vi "短信通知设置.vi"() -> ()   [LabVIEW 2017]
uses:
  <vilib>/Utility/xml.llb/Write to XML File(string).vi
panel:
  in  "通讯录菜单":enum16{"添加", "删除"}(ring)
  in  "联系人数组":cluster{"姓名":string, "手机号":string}[](array[cluster])
  in  "密码":string
  in  "短信通道":string
  in  "员工编号":string
  in  "企业编号":string
  in  "确定":bool
  in  "取消":bool
  in  "添加联系人":bool
  in  "通讯录":i32(listbox)
  # "登录信息"
  # "通讯录"
  # "* 短信通知功能需用户自行开通，详询对接平台 http://www.c123.com/"
  # "* 通讯录表格中右键菜单添加或删除联系人"
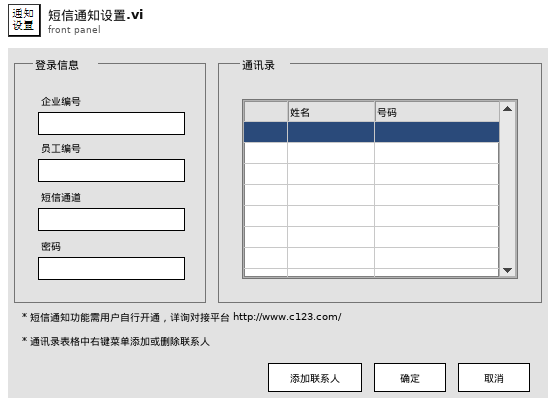
[diagram p1: front panel]
types:
  T1 = enum32{"Invalid", "Standard", "Closed", "Hidden", "Minimized", "Maximized"}
  T2 = cluster{"企业编号":string, "员工编号":string, "通道号":string, "密码":string, "联系人数组":cluster{"姓名":string, "手机号":string}[]}
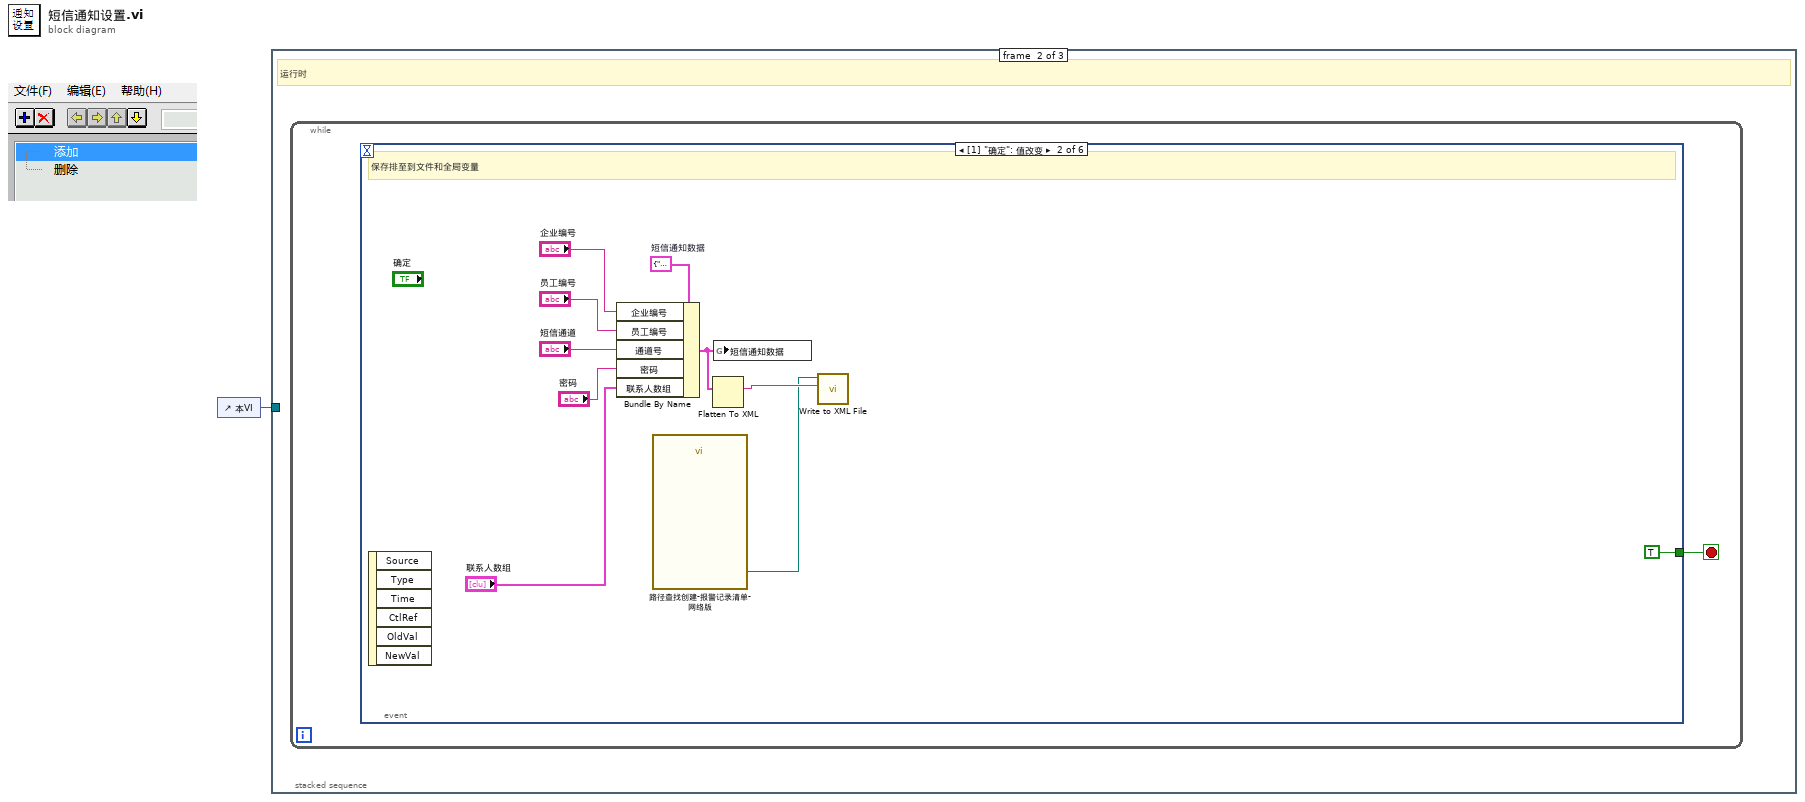
[diagram p0: block diagram]
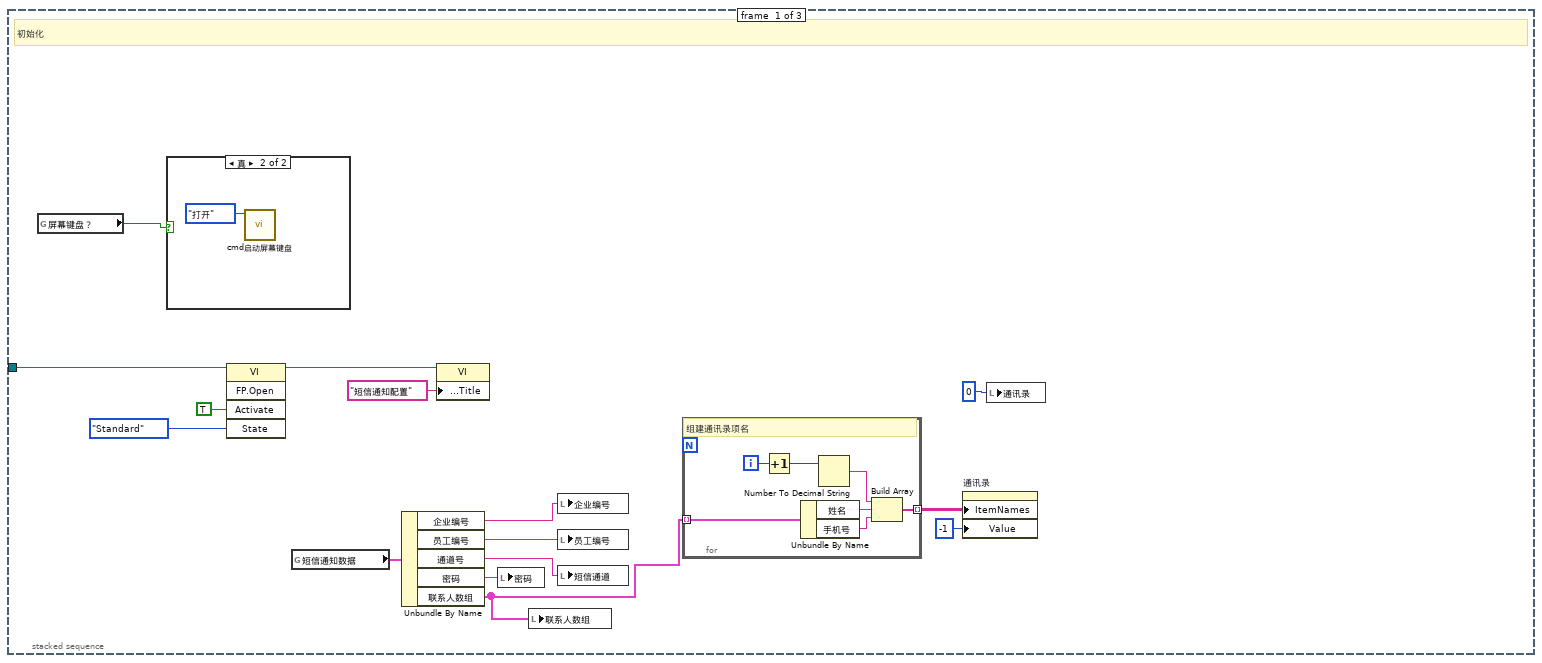
[diagram p2: hidden frame]
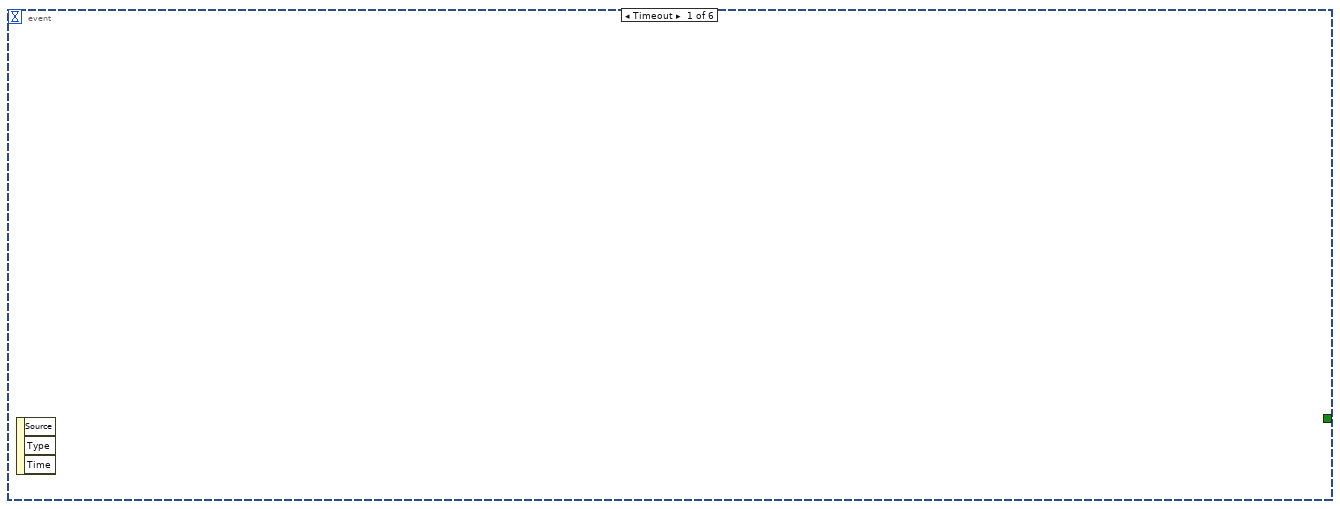
[diagram p4: hidden frame]
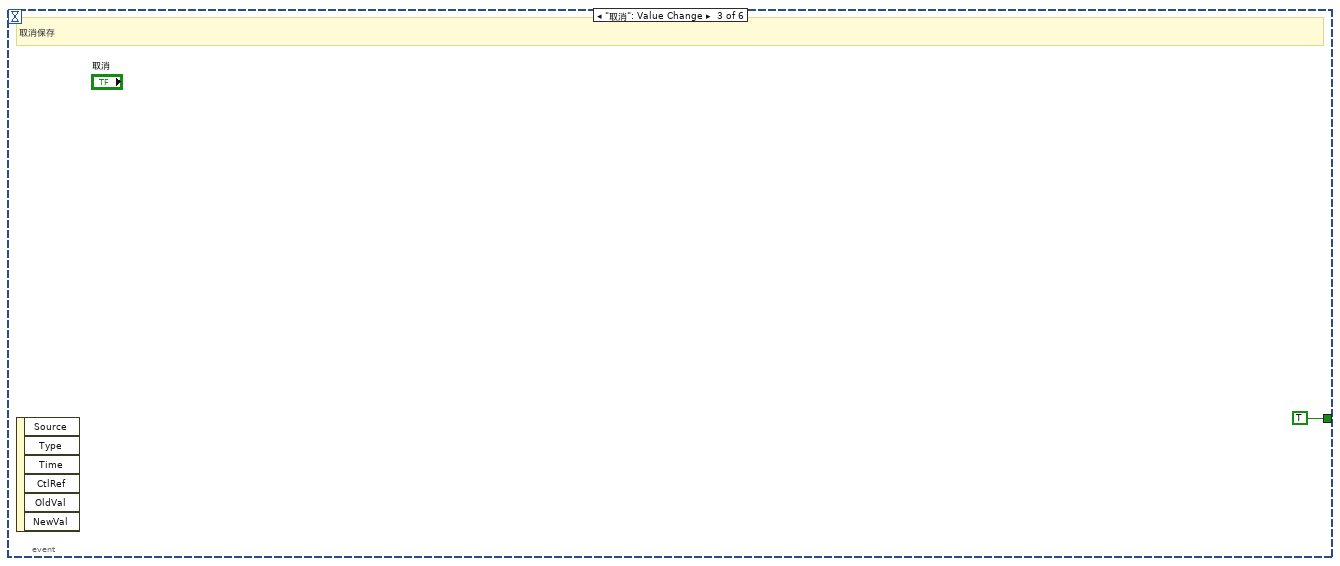
[diagram p5: hidden frame]
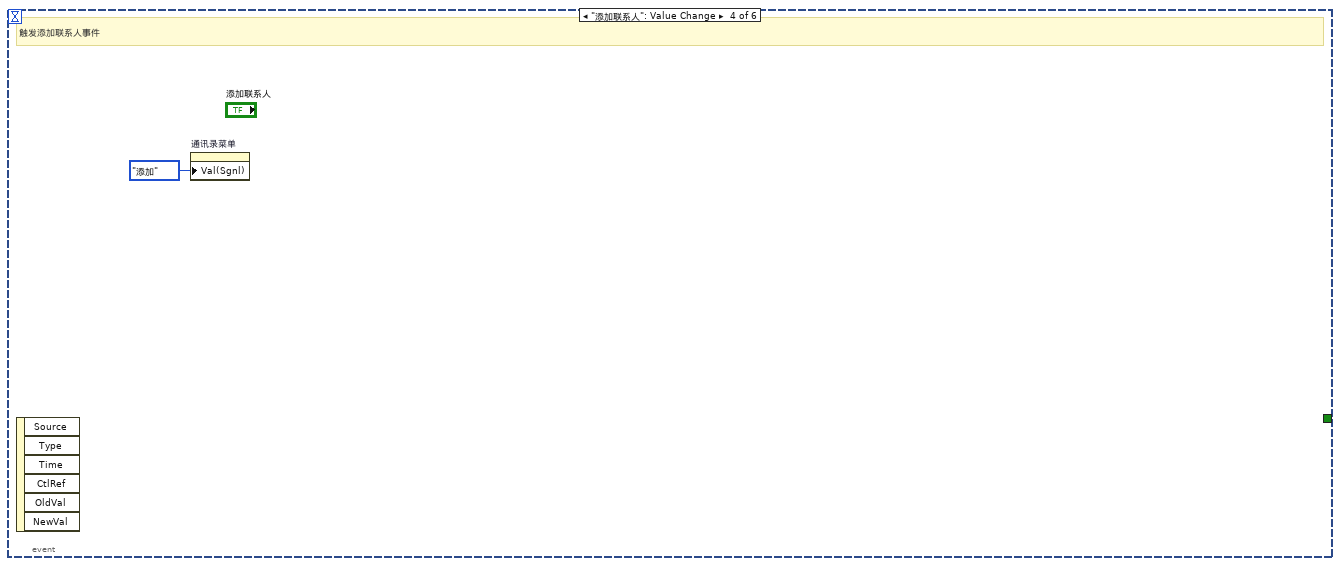
[diagram p6: hidden frame]
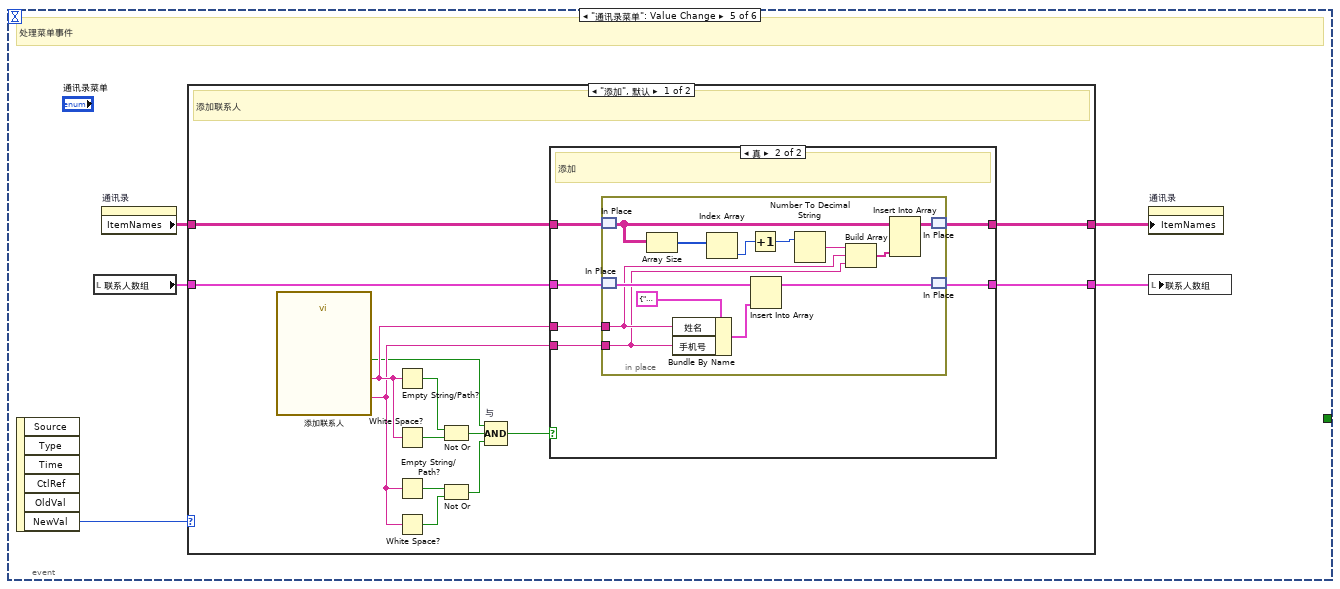
[diagram p7: hidden frame]
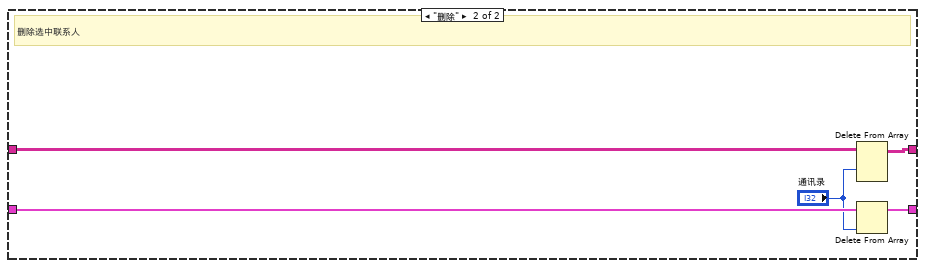
[diagram p9: hidden frame]
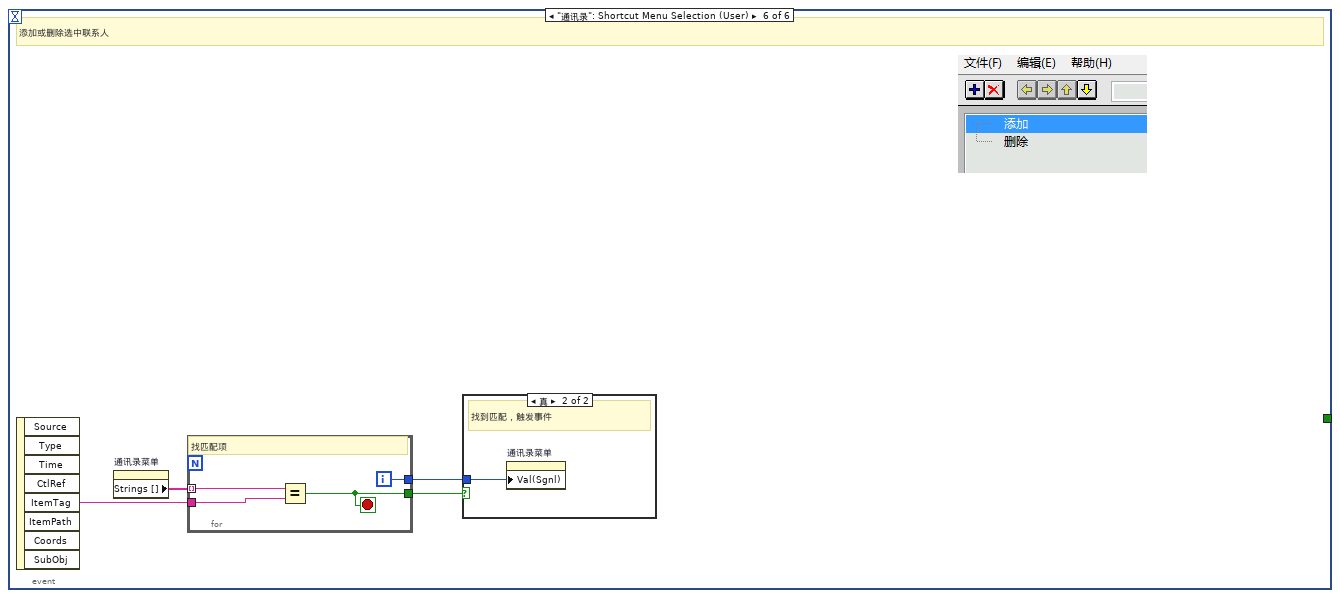
[diagram p10: hidden frame]
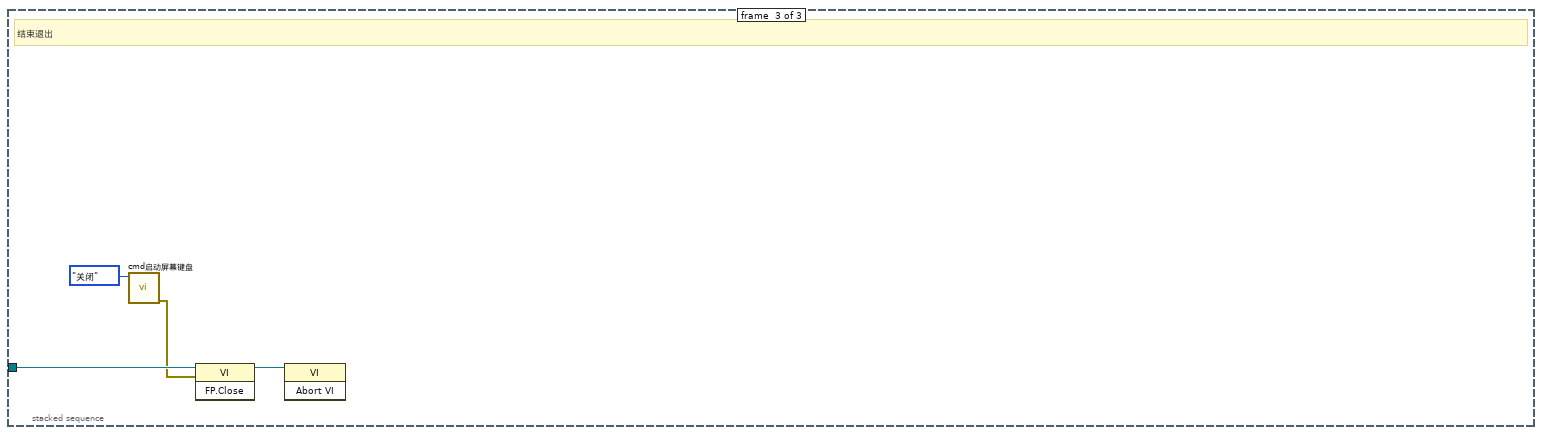
[diagram p12: hidden frame]
diagram:
  n1 = control-ref of="本VI"() -> (w1:refnum<vi>)
  n2 = stacked-sequence {
    tunnel: w1 -> [w7 _ w95]
    frame #0 {
      # "初始化"
      n3 = global read "全局变量-35点监测.vi" "屏幕键盘？"() -> (w2:bool)
      n4 = case shown="真" w2 {
        frame False {
        }
        frame True {
          n5 = call "cmd启动屏幕键盘.vi"("软键盘开关"=enum16{"关闭", "打开"}."打开") -> ()  [unwired: 9 in, 2 out]
        }
      }
      n6 = invoke class="VI" method="FP.Open"(reference=w7, "Activate"=TRUE ("激活？"), "State"=T1."Standard" ("状态")) -> (reference out=w5:refnum<vi>)  [unwired: 2 in, 4 out]
      n7 = global read "全局变量-35点监测.vi" "短信通知数据"() -> (w16:T2)
      n8 = Unbundle By Name(w16) -> ("企业编号"=w15:string, "员工编号"=w14:string, "通道号"=w13:string, "密码"=w12:string, "联系人数组"=w11:cluster{"姓名":string, "手机号":string}[])
      n9 = property class="VI"(reference=w5, "Front Panel.Title"="短信通知配置" ("前面板窗口:标题")) -> ()  [unwired: 1 in, 2 out]
      n10 = local write "密码"(w12) -> ()
      n11 = local write "联系人数组"(w11) -> ()
      n12 = local write "企业编号"(w15) -> ()
      n13 = local write "员工编号"(w14) -> ()
      n14 = local write "短信通道"(w13) -> ()
      n15 = for {
        tunnel: w11 -> [w24] mode=indexing
        tunnel: [w21] -> w10 mode=indexing
        i -> [w20]
        # "组建通讯录项名"
        n16 = Increment(x=w20) -> (x+1=w18:i32)
        n17 = Unbundle By Name(w24) -> ("姓名"=w23:string, "手机号"=w22:string)
        n18 = Number To Decimal String(number=w18) -> (decimal integer string=w19:string)  [unwired: 1 in]
        n19 = Build Array(w19, w23, w22) -> (w21:string[])
      }
      n20 = property on="通讯录" class="MCListbox (严格)"("ItemNames"=w10, "Value"=-1 ("通讯录")) -> ()  [unwired: 2 in, 2 out]
      n21 = local write "通讯录"(0 ("通讯录")) -> ()
    }
    frame #1 {
      # "运行时"
      n22 = while {
        stop <- w25 stop-if-true
        n23 = event shown="[1] \"确定\": 值改变" {
          selector: _ -> [_ _ _ _ _ _]
          dyn-events: _ -> [_ _ _ _ _ _]
          timeout: _ -> [_ _ _ _ _ _]
          tunnel: [_ TRUE TRUE _ _ _] -> w25
          event Timeout {
            n24 = event-data() -> ()  [unwired: 1 in, 3 out]
          }
          event "确定": Value Change {
            w35 = T2 {"企业编号"="", "员工编号"="", "通道号"="", "密码"="", "联系人数组"=[]}  # 短信通知数据
            # "保存排至到文件和全局变量"
            n25 = event-data() -> ()  [unwired: 1 in, 6 out]
            n26 = Bundle By Name(cluster=w35, "企业编号"="企业编号", "员工编号"="员工编号", "通道号"="短信通道", "密码"="密码", "联系人数组"="联系人数组") -> (w27:T2)
            n27 = call "路径查找创建-报警记录清单-网络版.vi"() -> ("短信通知配置文件"=w28:path)  [unwired: 2 in, 13 out]
            n28 = Flatten To XML(anything=w27) -> (xml string=w29:string)
            n29 = global write "全局变量-35点监测.vi" "短信通知数据"(w27) -> ()
            n30 = call-poly <vilib>:"Write to XML File.vi"("XML Input"=w29, "XML File Path"=w28) -> ()  [unwired: 7 in, 3 out]
          }
          event "取消": Value Change {
            # "取消保存"
            n31 = event-data() -> ()  [unwired: 1 in, 6 out]
          }
          event "添加联系人": Value Change {
            # "触发添加联系人事件"
            n32 = event-data() -> ()  [unwired: 1 in, 6 out]
            n33 = property on="通讯录菜单" class="Enum (严格)"("Val(Sgnl)"=enum16{"添加", "删除"}."添加" ("值(信号)")) -> ()  [unwired: 2 in, 2 out]
          }
          event "通讯录菜单": Value Change {
            # "处理菜单事件"
            n34 = event-data() -> ("NewVal"=w42:enum16{"添加", "删除"})  [unwired: 1 in, 5 out]
            n35 = local read "联系人数组"() -> (w41:cluster{"姓名":string, "手机号":string}[])
            n36 = property on="通讯录" class="MCListbox (严格)"() -> ("ItemNames"=w39:string[][])  [unwired: 2 in, 2 out]
            n37 = case shown="\"添加\", 默认" w42 {
              tunnel: w41 -> [w56 w82]
              tunnel: [w55 w81] -> w40
              tunnel: w39 -> [w54 w80]
              tunnel: [w53 w79] -> w38
              frame "添加", Default {
                # "添加联系人"
                n38 = call "添加联系人"() -> ("手机号码"=w51:string, "姓名"=w52:string, "确定"=w49:bool)  [unwired: 16 in, 1 out]
                n39 = Empty String/Path?(string/path=w52) -> (empty?=w48:bool)
                n40 = White Space?(1:w52) -> (0:w47:bool)
                n41 = Empty String/Path?(string/path=w51) -> (empty?=w50:bool)
                n42 = White Space?(1:w51) -> (0:w46:bool)
                n43 = Not Or(1:w47, 2:w48) -> (0:w45:bool)
                n44 = Not Or(1:w46, 2:w50) -> (0:w44:bool)
                n45 = Compound Arithmetic op=AND "与"(w49, w45, w44) -> (w43:bool)
                n46 = case shown="真" w43 {
                  tunnel: w52 -> [_ w64]
                  tunnel: w51 -> [_ w63]
                  tunnel: w56 -> [w58 w62]
                  tunnel: [w58 w61] -> w55
                  tunnel: w54 -> [w57 w60]
                  tunnel: [w57 w59] -> w53
                  frame False {
                    # "取消"
                  }
                  frame True {
                    # "添加"
                    n47 = in-place {
                      in-place-border: w64 -> [w68]
                      in-place-border: w63 -> [w67]
                      n48 = in-place-match #1(w60) -> (w72:string[][])
                      n49 = in-place-match #2(w62) -> (w77:cluster{"姓名":string, "手机号":string}[])
                      n50 = Array Size(array=w72) -> (size(s)=w71:i32[])
                      n51 = Bundle By Name(cluster=cluster{"姓名":string, "手机号":string} {"姓名"="", "手机号"=""} ("新元素/子数组"), "姓名"=w68, "手机号"=w67) -> (w73:cluster{"姓名":string, "手机号":string})
                      n52 = Index Array(array=w71) -> (element=w70:i32)  [unwired: 1 in]
                      n53 = Increment(x=w70) -> (x+1=w65:i32)
                      n54 = Insert Into Array(array=w77, new element=w73) -> (w76:cluster{"姓名":string, "手机号":string}[])  [unwired: 1 in]
                      n55 = Number To Decimal String(number=w65) -> (decimal integer string=w69:string)  [unwired: 1 in]
                      n56 = Build Array(w69, w68, w67) -> (w66:string[])
                      n57 = Insert Into Array(array=w72, new element=w66) -> (w75:string[][])  [unwired: 2 in]
                      n58 = in-place-match #1(w75) -> (w59:string[][])
                      n59 = in-place-match #2(w76) -> (w61:cluster{"姓名":string, "手机号":string}[])
                    }
                  }
                }
              }
              frame "删除" {
                # "删除选中联系人"
                n60 = Delete From Array(array=w80, index (row)="通讯录") -> (array with subset deleted=w79:string[][])  [unwired: 2 in, 1 out]
                n61 = Delete From Array(array=w82, index="通讯录") -> (array with subset deleted=w81:cluster{"姓名":string, "手机号":string}[])  [unwired: 1 in, 1 out]
              }
            }
            n62 = property on="通讯录" class="MCListbox (严格)"("ItemNames"=w38) -> ()  [unwired: 2 in, 2 out]
            n63 = local write "联系人数组"(w40) -> ()
          }
          event "通讯录": Shortcut Menu Selection (User) {
            # "添加或删除选中联系人"
            n64 = event-data() -> ("ItemTag"=w85:string)  [unwired: 1 in, 7 out]
            n65 = property on="通讯录菜单" class="Enum (严格)"() -> ("Strings []"=w86:string[])  [unwired: 2 in, 2 out]
            n66 = for {
              tunnel: w86 -> [w91] mode=indexing
              tunnel: w85 -> [w90]
              tunnel: [w89] -> w83
              tunnel: [w88] -> w84
              i -> [w88]
              stop <- w89 stop-if-true
              # "找匹配项"
              n67 = Equal?(x=w91, y=w90) -> (x = y?=w89:bool)
            }
            n68 = case shown="真" w83 {
              tunnel: w84 -> [_ w87]
              frame False {
                # "为未到匹配"
              }
              frame True {
                # "找到匹配，触发事件"
                n69 = property on="通讯录菜单" class="Enum (严格)"("Val(Sgnl)"=w87) -> ()  [unwired: 2 in, 2 out]
              }
            }
          }
        }
      }
    }
    frame #2 {
      # "结束退出"
      n70 = call "cmd启动屏幕键盘.vi"("软键盘开关"=enum16{"关闭", "打开"}."关闭") -> ("error out"=w92:errorcluster)  [unwired: 9 in, 1 out]
      n71 = invoke class="VI" method="FP.Close"(reference=w95, error in=w92) -> (reference out=w94:refnum<vi>)  [unwired: 1 in, 2 out]
      n72 = invoke class="VI" method="Abort VI"(reference=w94) -> ()  [unwired: 2 in, 3 out]
    }
  }
